vi "Save Rename VI.vi"(8 "error in":errorcluster, 9 "Rename":string, 10 "VI Ref":refnum<vi>) -> (0 "error out":errorcluster)   [LabVIEW 2025, in "_Rename.lvlib" / "_Rename.lvclass"]
uses:
  _Rename.lvclass
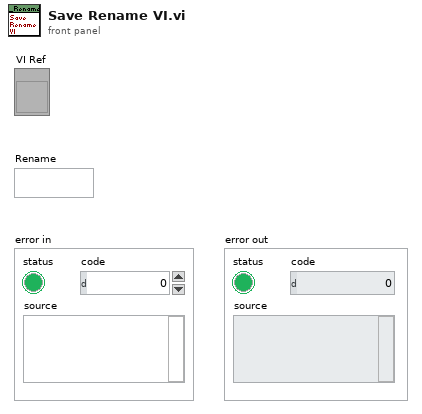
[diagram p1: front panel]
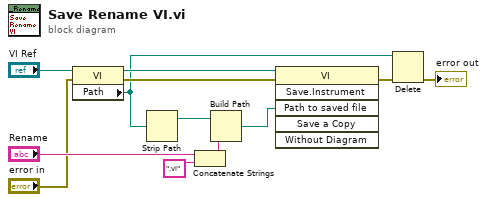
[diagram p0: block diagram]
diagram:
  n1 = property class="VI"(reference="VI Ref", error in="error in") -> (reference out=w7:refnum<vi>, error out=w8:errorcluster, "Path"=w3:path)
  n2 = Strip Path(path=w3) -> (stripped path=w11:path)  [unwired: 1 out]
  n3 = Concatenate Strings("Rename", ".vi" ("string")) -> (w9:string)
  n4 = Build Path(base path=w11, name or relative path=w9) -> (appended path=w12:path)
  n5 = invoke class="VI" method="Save.Instrument"(reference=w7, error in=w8, "Path to saved file"=w12) -> (error out=w2:errorcluster)  [unwired: 3 in, 5 out]
  n6 = Delete(path (use dialog)=w3, error in=w2) -> (error out=→"error out":errorcluster)  [unwired: 3 in, 2 out]
